vi "[ToBeTest-PC] Continuous Complete Measurament RT.vi"() -> ()   [LabVIEW 2014]
uses:
  <vilib>/FPGAPlugInAG/sbRIO-9636/niLvFpga_Open_sbRIO-9636.vi
  <vilib>/rvi/interface/common/dynamic/niFpgaDynamicAddResources.vi
  <vilib>/FPGAPlugInAG/Dynamic/niLvFpga_Reset_Dynamic.vi
  <vilib>/Utility/error.llb/Error Cluster From Error Code.vi
  <vilib>/rvi/errors/niLvFpgaAdjustHostInterfaceError.vi
  <vilib>/rvi/interface/common/niFpgaWaitOnOcc.vi
  <vilib>/FPGAPlugInAG/Dynamic/niLvFpga_Run_Dynamic.vi
  <vilib>/FPGAPlugInAG/Dynamic/niLvFpga_Abort_Dynamic.vi
  <vilib>/FPGAPlugInAG/Dynamic/niLvFpga_Close_Dynamic.vi
  <vilib>/rvi/interface/nirviOpenFPGA/nirviOpenFPGA.xnode
  FPGA Bitfiles/LaserDistanceSen_FPGATarget_N-ParametricDoub_oZd6Q4K0Aos.lvbitx
  FPGA Target/Test VIs/N-Parametric Double FFT Mesurament (MAX BIN DETECT) SLOW Test.vi
  <vilib>/rvi/interface/nirviMethod/nirviMethod.xnode
  <vilib>/rvi/interface/nirviReadWriteControl/nirviReadWriteControl.xnode
  <vilib>/rvi/interface/nirviCloseFPGA/nirviCloseFPGA.xnode
  <vilib>/rvi/errors/niLvFpgaMergeErrorWithErrorCode.vi
  <vilib>/rvi/interface/Simulation/niFpgaSimulationCallBeginRW.vi
  NiFpgaLv.dll
  <vilib>/Analysis/NI_AALBase.lvlib
  <vilib>/FPGAPlugInAG/Dynamic/niLvFpga_ConfigureFifo_Dynamic.vi
  <vilib>/FPGAPlugInAG/Dynamic/niLvFpga_StartFifo_Dynamic.vi
  <vilib>/FPGAPlugInAG/Dynamic/niLvFpga_ReadFifo_Dynamic.vi
panel:
  out "Standard deviation (m)":dbl format="%0.5f"
  out "cycle time":u32
  out "Distance (m) Plot":dbl(graph)
  in  "#signal for Mean":i32=3000
  out "Relative Standard Deviation":dbl format="%0.7f"
  out "Distance (m)":dbl format="%0.7f"
  in  "stop":bool
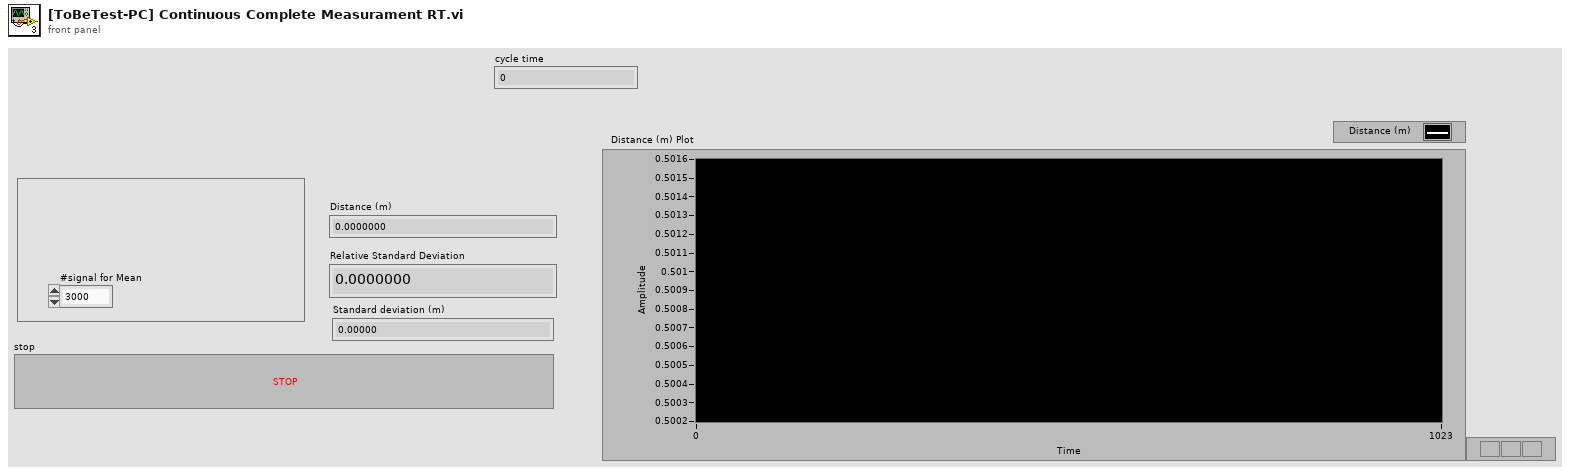
[diagram p1: front panel]
types:
  T1 = enum16{"None", "Hanning", "Hamming", "Blackman", "Blackman-Harris"}
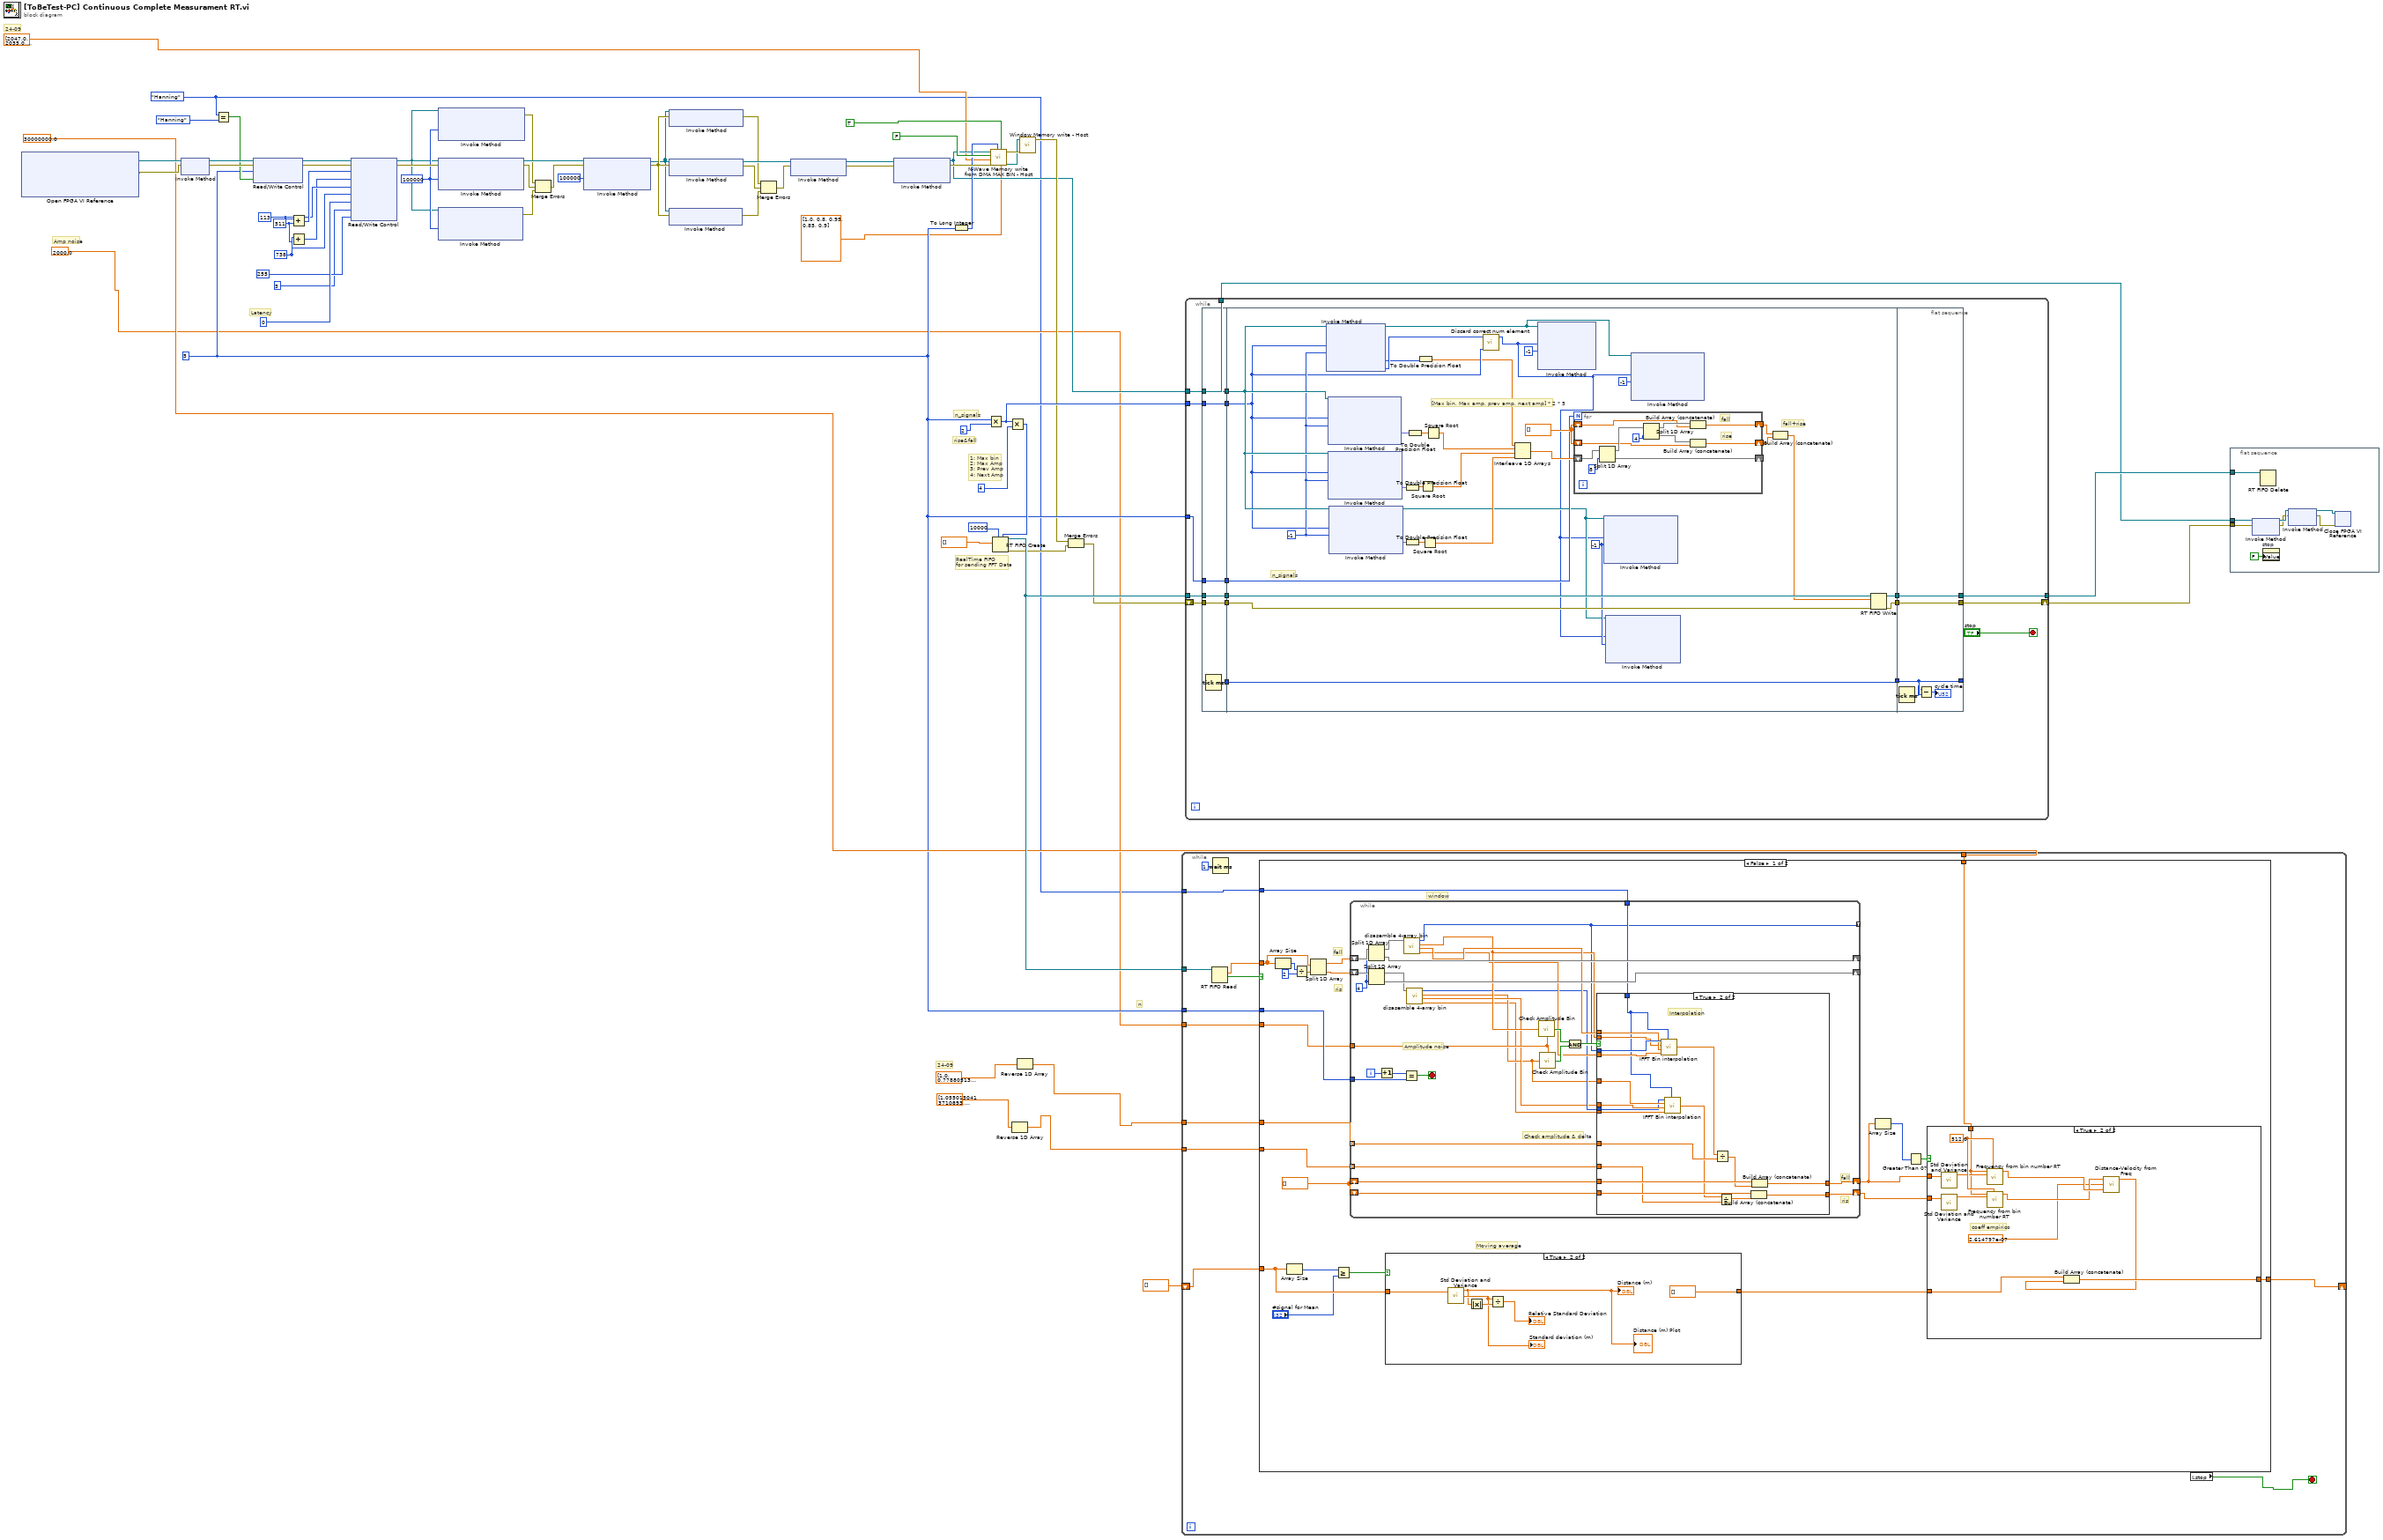
[diagram p0: block diagram]
diagram:
  w6 = T1."Hanning" ("Windowing")
  w62 = u32 738 ("lower limit 2")
  w64 = u32 113 ("lower limit 1")
  w25 = u32 5 ("#Signals")
  w43 = u32 100000 ("Requested Depth")
  w61 = u32 511 ("y")
  # "24-09"
  # "Latency"
  # "24-09"
  # "Amp noise"
  # "n_signals"
  # "rise&fall"
  # "1: Max bin\n2: Max Amp\n3: Prev Amp\n4: Next Amp"
  # "n"
  # "RealTime FIFO \nfor sending FFT Data"
  n1 = xnode "Open FPGA VI Reference"() -> ("FPGA VI Reference Out"=w56:refnum<k20>, "error out"=w55:errorcluster)  [unwired: 2 in]
  n2 = xnode "Invoke Method"("FPGA VI Reference In"=w56, "error in"=w55) -> ("FPGA VI Reference Out"=w53:refnum<k20>, "error out"=w54:errorcluster)
  n3 = Equal?(x=w6, y=T1."Hanning" ("Windowing")) -> (x = y?=w46:bool)
  n4 = xnode "Read/Write Control"("FPGA VI Reference In"=w53, "error in"=w54, "n"=w25, "Hanning window"=w46) -> ("FPGA VI Reference Out"=w52:refnum<k20>, "error out"=w51:errorcluster)
  n5 = Add(x=w64, y=w61) -> (x+y=w65:u32)
  n6 = Add(x=w62, y=w61) -> (x+y=w63:u32)
  n7 = xnode "Read/Write Control"("FPGA VI Reference In"=w52, "error in"=w51, "upper limit 1"=w65, "upper limit 2"=w63, "lower limit 1"=w64, "lower limit 2"=w62, "Latency points"=u32 0 ("Initial Latency points"), "First bin"=5 ("first bin"), "Last bin"=255 ("last bin")) -> ("FPGA VI Reference Out"=w23:refnum<k20>, "error out"=w60:errorcluster)
  n8 = xnode "Invoke Method"("FPGA VI Reference In"=w23, "Requested Depth"=w43) -> ("error out"=w42:errorcluster)  [unwired: 1 in, 2 out]
  n9 = xnode "Invoke Method"("FPGA VI Reference In"=w23, "error in"=w60, "Requested Depth"=w43) -> ("FPGA VI Reference Out"=w57:refnum<k20>, "error out"=w41:errorcluster)  [unwired: 1 out]
  n10 = xnode "Invoke Method"("FPGA VI Reference In"=w23, "Requested Depth"=w43) -> ("error out"=w40:errorcluster)  [unwired: 1 in, 2 out]
  n11 = Merge Errors(w42, w41, w40) -> (w39:errorcluster)
  n12 = xnode "Invoke Method"("FPGA VI Reference In"=w57, "error in"=w39, "Requested Depth"=u32 100000) -> ("FPGA VI Reference Out"=w31:refnum<k20>, "error out"=w32:errorcluster)  [unwired: 1 out]
  n13 = xnode "Invoke Method"("FPGA VI Reference In"=w31, "error in"=w32) -> ("error out"=w30:errorcluster)  [unwired: 1 out]
  n14 = xnode "Invoke Method"("FPGA VI Reference In"=w31, "error in"=w32) -> ("FPGA VI Reference Out"=w35:refnum<k20>, "error out"=w36:errorcluster)
  n15 = xnode "Invoke Method"("FPGA VI Reference In"=w31, "error in"=w32) -> ("error out"=w37:errorcluster)  [unwired: 1 out]
  n16 = Merge Errors(w30, w36, w37) -> (w38:errorcluster)
  n17 = xnode "Invoke Method"("FPGA VI Reference In"=w35, "error in"=w38) -> ("FPGA VI Reference Out"=w34:refnum<k20>, "error out"=w33:errorcluster)
  n18 = xnode "Invoke Method"("FPGA VI Reference In"=w34, "error in"=w33) -> ("FPGA VI Reference Out"=w10:refnum<k20>, "error out"=w15:errorcluster)  [unwired: 1 in]
  n19 = To Long Integer(number=w25) -> (32bit integer=w12:i32)
  n20 = Multiply(x=w25, y=u32 2 ("elements in array (1)")) -> (x*y=w26:u32)
  n21 = call "N-Wave Memory write from DMA MAX BIN - Host.vi"("Triangular Multiply Factor"=dbl[] [1.0, 0.8, 0.95, 0.85, 0.9], "Enable triangular scaling"=TRUE, "n"=w12, "error in"=w15, "Custom Triangular Signal (fal-ris)"=dbl[] [2047.0, 2035.0, 2022.0, 2010.0, 1997.0, 1985.0, 1972.0, 1960.0, 1948.0, 1935.0, 1923.0, 1911.0, 1899.0, 1886.0, 1874.0, 1862.0, 1850.0, 1838.0, 1825.0, 1813.0, 1801.0, 1789.0, 1777.0, 1765.0, 1753.0, 1741.0, 1729.0, 1717.0, 1705.0, 1693.0, 1681.0, 1669.0, 1657.0, 1645.0, 1634.0, 1622.0, 1610.0, 1598.0, 1586.0, 1575.0, 1563.0, 1551.0, 1540.0, 1528.0, 1516.0, 1505.0, 1493.0, 1481.0, 1470.0, 1458.0, 1447.0, 1435.0, 1424.0, 1412.0, 1401.0, 1389.0, 1378.0, 1366.0, 1355.0, 1344.0, 1332.0, 1321.0, 1310.0, 1298.0, 1287.0, 1276.0, 1265.0, 1253.0, 1242.0, 1231.0, 1220.0, 1209.0, 1198.0, 1186.0, 1175.0, 1164.0, 1153.0, 1142.0, 1131.0, 1120.0, 1109.0, 1098.0, 1087.0, 1076.0, 1065.0, 1055.0, 1044.0, 1033.0, 1022.0, 1011.0, 1000.0, 990.0, 979.0, 968.0, 958.0, 947.0, 936.0, 926.0, 915.0, 904.0, 894.0, 883.0, 873.0, 862.0, 852.0, 841.0, 831.0, 820.0, 810.0, 799.0, 789.0, 778.0, 768.0, 758.0, 747.0, 738.0, 727.0, 719.0, 712.0, 706.0, 700.0, 693.0, 687.0, 680.0, 674.0, 668.0, 661.0, 655.0, 648.0, 642.0, 636.0, 629.0, 623.0, 617.0, 610.0, 604.0, 598.0, 591.0, 584.0, 577.0, 569.0, 560.0, 552.0, 545.0, 538.0, 531.0, 525.0, 519.0, 512.0, 506.0, 500.0, 494.0, 488.0, 482.0, 476.0, 470.0, 464.0, 458.0, 452.0, 446.0, 436.0, 430.0, 424.0, 418.0, 412.0, 406.0, 400.0, 394.0, 388.0, 382.0, 376.0, 370.0, 364.0, 358.0, 352.0, 346.0, 338.0, 332.0, 325.0, 319.0, 313.0, 307.0, 301.0, 295.0, 290.0, 284.0, 278.0, 272.0, 267.0, 261.0, 255.0, 249.0, 244.0, 238.0, 232.0, 227.0, 221.0, 215.0, 209.0, 204.0, 198.0, 192.0, 187.0, 181.0, 175.0, 170.0, 164.0, 158.0, 153.0, 147.0, 141.0, 136.0, 130.0, 124.0, 119.0, 113.0, 108.0, 102.0, 96.0, 91.0, 85.0, 79.0, 74.0, 68.0, 62.0, 57.0, 51.0, 45.0, 39.0, 34.0, 28.0, 22.0, 16.0, 11.0, 5.0, 0.0, -6.0, -11.0, -17.0, -22.0, -28.0, -33.0, -39.0, -44.0, -50.0, -55.0, -61.0, -66.0, -72.0, -77.0, -83.0, -88.0, -94.0, -99.0, -105.0, -110.0, -116.0, -121.0, -127.0, -132.0, -137.0, -143.0, -148.0, -154.0, -159.0, -165.0, -170.0, -176.0, -181.0, -186.0, -192.0, -197.0, -203.0, -208.0, -214.0, -219.0, -224.0, -230.0, -235.0, -241.0, -246.0, -251.0, -257.0, -262.0, -268.0, -273.0, -278.0, -284.0, -289.0, -295.0, -300.0, -305.0, -311.0, -316.0, -321.0, -327.0, -332.0, -337.0, -343.0, -348.0, -354.0, -359.0, -364.0, -370.0, -375.0, -380.0, -386.0, -391.0, -397.0, -402.0, -407.0, -413.0, -418.0, -423.0, -429.0, -434.0, -439.0, -445.0, -450.0, -455.0, -461.0, -466.0, -471.0, -477.0, -482.0, -487.0, -493.0, -498.0, -503.0, -509.0, -514.0, -519.0, -525.0, -530.0, -535.0, -540.0, -546.0, -551.0, -556.0, -562.0, -567.0, -572.0, -578.0, -583.0, -588.0, -593.0, -599.0, -604.0, -609.0, -615.0, -620.0, -625.0, -630.0, -636.0, -641.0, -646.0, -651.0, -657.0, -662.0, -667.0, -673.0, -678.0, -683.0, -688.0, -694.0, -699.0, -704.0, -709.0, -715.0, -720.0, -725.0, -730.0, -736.0, -741.0, -746.0, -751.0, -757.0, -762.0, -767.0, -772.0, -778.0, -783.0, -788.0, -793.0, -799.0, -804.0, -809.0, -814.0, -820.0, -825.0, -830.0, -835.0, -841.0, -846.0, -851.0, -856.0, -862.0, -867.0, -872.0, -877.0, -883.0, -888.0, -893.0, -898.0, -903.0, -909.0, -914.0, -919.0, -924.0, -930.0, -935.0, -940.0, -945.0, -951.0, -956.0, -961.0, -966.0, -971.0, -977.0, -982.0, -987.0, -992.0, -998.0, -1003.0, -1008.0, -1013.0, -1018.0, -1024.0, -1029.0, -1034.0, -1039.0, -1045.0, -1050.0, -1055.0, -1060.0, -1065.0, -1071.0, -1076.0, -1081.0, -1086.0, -1092.0, -1097.0, -1102.0, -1107.0, -1112.0, -1118.0, -1123.0, -1128.0, -1133.0, -1138.0, -1144.0, -1149.0, -1154.0, -1159.0, -1165.0, -1170.0, -1175.0, -1180.0, -1185.0, -1191.0, -1196.0, -1201.0, -1206.0, -1211.0, -1217.0, -1222.0, -1227.0, -1232.0, -1237.0, -1243.0, -1248.0, -1253.0, -1258.0, -1263.0, -1269.0, -1274.0, -1279.0, -1284.0, -1289.0, -1295.0, -1300.0, -1305.0, -1310.0, -1315.0, -1321.0, -1326.0, -1331.0, -1336.0, -1341.0, -1347.0, -1352.0, -1357.0, -1362.0, -1367.0, -1373.0, -1378.0, -1383.0, -1388.0, -1393.0, -1399.0, -1404.0, -1409.0, -1414.0, -1419.0, -1425.0, -1430.0, -1435.0, -1440.0, -1445.0, -1450.0, -1456.0, -1461.0, -1466.0, -1471.0, -1476.0, -1482.0, -1487.0, -1492.0, -1497.0, -1502.0, -1508.0, -1513.0, -1518.0, -1523.0, -1528.0, -1534.0, -1539.0, -1544.0, -1549.0, -1554.0, -1560.0, -1565.0, -1570.0, -1575.0, -1580.0, -1586.0, -1591.0, -1596.0, -1601.0, -1606.0, -1612.0, -1617.0, -1622.0, -1627.0, -1632.0, -1637.0, -1643.0, -1648.0, -1653.0, -1658.0, -1663.0, -1669.0, -1674.0, -1679.0, -1684.0, -1689.0, -1695.0, -1700.0, -1705.0, -1710.0, -1715.0, -1721.0, -1726.0, -1731.0, -1736.0, -1741.0, -1747.0, -1752.0, -1757.0, -1762.0, -1767.0, -1773.0, -1778.0, -1783.0, -1788.0, -1793.0, -1799.0, -1804.0, -1809.0, -1814.0, -1819.0, -1825.0, -1830.0, -1835.0, -1840.0, -1845.0, -1851.0, -1856.0, -1861.0, -1866.0, -1871.0, -1876.0, -1882.0, -1887.0, -1892.0, -1897.0, -1902.0, -1908.0, -1913.0, -1918.0, -1923.0, -1928.0, -1934.0, -1939.0, -1944.0, -1949.0, -1954.0, -1960.0, -1965.0, -1970.0, -1975.0, -1980.0, -1986.0, -1991.0, -1996.0, -2001.0, -2006.0, -2012.0, -2017.0, -2022.0, -2027.0, -2032.0, -2038.0, -2043.0, -2048.0, -2047.0, -2037.0, -2027.0, -2017.0, -2007.0, -1997.0, -1987.0, -1977.0, -1967.0, -1957.0, -1947.0, -1937.0, -1927.0, -1917.0, -1907.0, -1897.0, -1888.0, -1878.0, -1868.0, -1858.0, -1848.0, -1838.0, -1828.0, -1819.0, -1809.0, -1799.0, -1789.0, -1780.0, -1770.0, -1760.0, -1750.0, -1741.0, -1731.0, -1721.0, -1712.0, -1702.0, -1692.0, -1683.0, -1673.0, -1663.0, -1654.0, -1644.0, -1635.0, -1625.0, -1615.0, -1606.0, -1596.0, -1587.0, -1577.0, -1568.0, -1558.0, -1549.0, -1539.0, -1530.0, -1520.0, -1511.0, -1501.0, -1492.0, -1483.0, -1473.0, -1464.0, -1454.0, -1445.0, -1436.0, -1426.0, -1417.0, -1408.0, -1398.0, -1389.0, -1380.0, -1371.0, -1361.0, -1352.0, -1343.0, -1334.0, -1324.0, -1315.0, -1306.0, -1297.0, -1288.0, -1278.0, -1269.0, -1260.0, -1251.0, -1242.0, -1233.0, -1224.0, -1215.0, -1205.0, -1196.0, -1187.0, -1178.0, -1169.0, -1160.0, -1151.0, -1142.0, -1133.0, -1124.0, -1115.0, -1106.0, -1097.0, -1088.0, -1080.0, -1071.0, -1062.0, -1053.0, -1044.0, -1035.0, -1026.0, -1017.0, -1009.0, -1000.0, -991.0, -982.0, -973.0, -965.0, -953.0, -944.0, -935.0, -920.0, -906.0, -889.0, -871.0, -854.0, -842.0, -834.0, -826.0, -818.0, -810.0, -802.0, -794.0, -786.0, -778.0, -770.0, -762.0, -754.0, -746.0, -739.0, -731.0, -723.0, -715.0, -707.0, -699.0, -690.0, -682.0, -672.0, -661.0, -651.0, -639.0, -627.0, -616.0, -606.0, -598.0, -591.0, -584.0, -577.0, -570.0, -563.0, -556.0, -549.0, -542.0, -535.0, -528.0, -520.0, -513.0, -506.0, -499.0, -492.0, -485.0, -478.0, -471.0, -464.0, -457.0, -451.0, -444.0, -437.0, -430.0, -423.0, -416.0, -409.0, -400.0, -390.0, -382.0, -373.0, -364.0, -356.0, -349.0, -343.0, -336.0, -330.0, -323.0, -317.0, -310.0, -304.0, -297.0, -291.0, -284.0, -278.0, -271.0, -265.0, -258.0, -252.0, -245.0, -239.0, -232.0, -226.0, -219.0, -213.0, -207.0, -200.0, -194.0, -187.0, -181.0, -175.0, -168.0, -162.0, -156.0, -149.0, -143.0, -136.0, -128.0, -121.0, -114.0, -107.0, -100.0, -93.0, -87.0, -80.0, -74.0, -68.0, -62.0, -56.0, -50.0, -44.0, -38.0, -32.0, -26.0, -20.0, -14.0, -8.0, -2.0, 5.0, 11.0, 17.0, 23.0, 29.0, 35.0, 41.0, 47.0, 53.0, 59.0, 65.0, 70.0, 76.0, 82.0, 88.0, 94.0, 100.0, 106.0, 112.0, 118.0, 124.0, 130.0, 136.0, 142.0, 148.0, 154.0, 161.0, 167.0, 174.0, 180.0, 186.0, 192.0, 198.0, 204.0, 210.0, 215.0, 221.0, 227.0, 233.0, 238.0, 244.0, 250.0, 255.0, 261.0, 267.0, 273.0, 278.0, 284.0, 290.0, 295.0, 301.0, 307.0, 312.0, 318.0, 324.0, 329.0, 335.0, 341.0, 346.0, 352.0, 358.0, 363.0, 369.0, 374.0, 380.0, 386.0, 391.0, 397.0, 402.0, 408.0, 414.0, 419.0, 425.0, 430.0, 436.0, 441.0, 447.0, 453.0, 458.0, 464.0, 470.0, 475.0, 481.0, 487.0, 493.0, 499.0, 504.0, 510.0, 516.0, 521.0, 527.0, 532.0, 538.0, 543.0, 549.0, 554.0, 560.0, 565.0, 571.0, 576.0, 582.0, 587.0, 593.0, 598.0, 604.0, 609.0, 614.0, 620.0, 625.0, 631.0, 636.0, 642.0, 647.0, 653.0, 658.0, 663.0, 669.0, 674.0, 680.0, 685.0, 691.0, 696.0, 701.0, 707.0, 712.0, 718.0, 723.0, 728.0, 734.0, 739.0, 745.0, 750.0, 755.0, 761.0, 766.0, 772.0, 777.0, 782.0, 788.0, 793.0, 798.0, 804.0, 809.0, 815.0, 820.0, 826.0, 831.0, 837.0, 842.0, 847.0, 853.0, 858.0, 863.0, 869.0, 874.0, 880.0, 885.0, 890.0, 895.0, 901.0, 906.0, 911.0, 917.0, 922.0, 927.0, 933.0, 938.0, 943.0, 948.0, 954.0, 959.0, 964.0, 970.0, 975.0, 980.0, 985.0, 991.0, 996.0, 1001.0, 1006.0, 1012.0, 1017.0, 1022.0, 1027.0, 1033.0, 1038.0, 1043.0, 1048.0, 1054.0, 1059.0, 1064.0, 1069.0, 1075.0, 1080.0, 1085.0, 1090.0, 1096.0, 1101.0, 1106.0, 1111.0, 1116.0, 1122.0, 1127.0, 1132.0, 1137.0, 1143.0, 1148.0, 1153.0, 1158.0, 1163.0, 1169.0, 1174.0, 1179.0, 1184.0, 1190.0, 1195.0, 1200.0, 1205.0, 1211.0, 1216.0, 1221.0, 1226.0, 1231.0, 1237.0, 1242.0, 1247.0, 1252.0, 1257.0, 1262.0, 1268.0, 1273.0, 1278.0, 1283.0, 1288.0, 1293.0, 1298.0, 1304.0, 1309.0, 1314.0, 1319.0, 1324.0, 1329.0, 1334.0, 1340.0, 1345.0, 1350.0, 1355.0, 1360.0, 1365.0, 1370.0, 1375.0, 1381.0, 1386.0, 1391.0, 1396.0, 1401.0, 1406.0, 1411.0, 1416.0, 1421.0, 1427.0, 1432.0, 1437.0, 1442.0, 1447.0, 1452.0, 1457.0, 1462.0, 1467.0, 1472.0, 1478.0, 1483.0, 1488.0, 1493.0, 1498.0, 1503.0, 1508.0, 1513.0, 1518.0, 1523.0, 1528.0, 1534.0, 1539.0, 1544.0, 1549.0, 1554.0, 1559.0, 1564.0, 1569.0, 1574.0, 1579.0, 1584.0, 1589.0, 1595.0, 1600.0, 1605.0, 1610.0, 1615.0, 1620.0, 1625.0, 1630.0, 1635.0, 1640.0, 1645.0, 1650.0, 1655.0, 1660.0, 1666.0, 1671.0, 1676.0, 1681.0, 1686.0, 1691.0, 1696.0, 1701.0, 1706.0, 1711.0, 1716.0, 1721.0, 1726.0, 1731.0, 1736.0, 1741.0, 1746.0, 1751.0, 1757.0, 1762.0, 1767.0, 1772.0, 1777.0, 1782.0, 1787.0, 1792.0, 1797.0, 1802.0, 1807.0, 1812.0, 1817.0, 1822.0, 1827.0, 1832.0, 1837.0, 1842.0, 1847.0, 1852.0, 1857.0, 1862.0, 1867.0, 1872.0, 1877.0, 1883.0, 1888.0, 1893.0, 1898.0, 1903.0, 1908.0, 1913.0, 1918.0, 1923.0, 1928.0, 1933.0, 1938.0, 1943.0, 1948.0, 1953.0, 1958.0, 1963.0, 1968.0, 1973.0, 1978.0, 1983.0, 1988.0, 1993.0, 1998.0, 2003.0, 2008.0, 2013.0, 2018.0, 2023.0, 2028.0, 2033.0, 2038.0, 2043.0, 2048.0] ("appended array"), "Triangolo dritto?"=FALSE, "FPGA VI Reference In"=w10) -> ("FPGA VI Reference Out"=w11:refnum<k20>, "error out"=w16:errorcluster)  [unwired: 2 in, 1 out]
  n22 = Multiply(x=w26, y=u32 4 ("elements in array (1)")) -> (x*y=w27:u32)
  n23 = RT FIFO Create(1:dbl[] [] ("first subarray"), 4:u32 10000 ("size (10)"), 6:w27) -> (8:w49:refnum<k33>, 11:w19:errorcluster)  [unwired: 5 in, 1 out]
  n24 = Reverse 1D Array(array=dbl[] [1.0550150413710893, 0.8807744280543515, 1.0096480344577006, 0.9233799836458207, 0.9653106595082892] ("mean factor 2")) -> (reversed array=w1:dbl[])
  n25 = Reverse 1D Array(array=dbl[] [1.0, 0.7788051374952276, 0.9586568902543302, 0.8395566206470091, 0.903068410955916] ("mean factor 1")) -> (reversed array=w3:dbl[])
  n26 = call "Window Memory write - Host.vi"("error in"=w16, "FPGA VI Reference In"=w11) -> ("error out"=w17:errorcluster)  [unwired: 7 in, 2 out]
  n27 = Merge Errors(w17, w19) -> (w18:errorcluster)
  n28 = while {
    tunnel: w49 -> [w78]
    tunnel: w6 -> [w75]
    tunnel: w25 -> [w74]
    shift-right: [w72] -> _
    shift-left: dbl[] [] ("appended array") -> [w73]
    tunnel: 30000000.0 -> [w71]
    tunnel: w3 -> [w70]
    tunnel: w1 -> [w69]
    tunnel: 2000.0 ("Threshold Amp") -> [w68]
    stop <- w66 stop-if-true
    n29 = RT FIFO Read(0:w78) -> (9:w76:dbl[], 10:w77:bool)  [unwired: 3 in, 3 out]
    n30 = Wait (ms)(milliseconds to wait=u32 1) -> ()  [unwired: 1 out]
    n31 = case shown="False" w77 {
      tunnel: w76 -> [w101 _]
      tunnel: w75 -> [w100 _]
      tunnel: w74 -> [w97 _]
      tunnel: w73 -> [w90 w173]
      tunnel: [w88 w173] -> w72
      tunnel: w71 -> [w79 _]
      tunnel: w70 -> [w87 _]
      tunnel: w69 -> [w86 _]
      tunnel: w68 -> [w85 _]
      frame False {
        w96 = dbl[] [] ("appended array")
        # "Moving average"
        # "window"
        # "ris"
        # "fall"
        n32 = Array Size(array=w101) -> (size(s)=w84:i32)
        n33 = Array Size(array=w90) -> (size(s)=w91:i32)
        n34 = Divide(x=w84, y=2) -> (x/y=w82:dbl)
        n35 = Split 1D Array(array=w101, index=w82) -> (first subarray=w98:dbl[], second subarray=w99:dbl[])
        n36 = Greater Or Equal?(x=w91, y="#signal for Mean") -> (x >= y?=w81:bool)
        n37 = while {
          shift-right: [w143] -> _
          shift-left: w98 -> [w151]
          shift-right: [w144] -> _
          shift-left: w99 -> [w150]
          tunnel: w100 -> [w139]
          tunnel: w97 -> [w148]
          shift-right: [w138] -> w95
          shift-left: w96 -> [w136]
          shift-right: [w137] -> w94
          shift-left: w96 -> [w135]
          tunnel: w87 -> [w134] mode=indexing
          tunnel: w86 -> [w133] mode=indexing
          tunnel: w85 -> [w132]
          tunnel: [w122] -> _ mode=indexing
          i -> [w145]
          stop <- w149 stop-if-true
          w147 = 4 ("x")
          # "ris"
          # "fall"
          # "Check amplitude & delta"
          # "Amplitude noise"
          n38 = Split 1D Array(array=w151, index=w147) -> (first subarray=w131:dbl[], second subarray=w143:dbl[])
          n39 = Split 1D Array(array=w150, index=w147) -> (first subarray=w130:dbl[], second subarray=w144:dbl[])
          n40 = Increment(x=w145) -> (x+1=w146:i32)
          n41 = Equal?(x=w146, y=w148) -> (x = y?=w149:bool)
          n42 = call "disasemble 4-array bin.vi"("4-Array Bin-Amp"=w131) -> ("Next Amp"=w127:dbl, "Prev amp"=w129:dbl, "Max amp"=w128:dbl, "Max bin"=w122:i32)  [unwired: 7 in]
          n43 = call "disasemble 4-array bin.vi"("4-Array Bin-Amp"=w130) -> ("Next Amp"=w123:dbl, "Prev amp"=w125:dbl, "Max amp"=w124:dbl, "Max bin"=w126:i32)  [unwired: 7 in]
          n44 = call "Check Amplitude Bin.vi"("Threshold Amp"=w132, "Max Amp"=w128) -> ("Check Amp Ok?"=w142:bool)  [unwired: 2 in]
          n45 = call "Check Amplitude Bin.vi"("Threshold Amp"=w132, "Max Amp"=w124) -> ("Check Amp Ok?"=w141:bool)  [unwired: 2 in]
          n46 = And(x=w142, y=w141) -> (x .and. y?=w140:bool)
          n47 = case shown="True" w140 {
            tunnel: w125 -> [_ w172]
            tunnel: w123 -> [_ w171]
            tunnel: w124 -> [_ w170]
            tunnel: w126 -> [_ w169]
            tunnel: w122 -> [_ w168]
            tunnel: w129 -> [_ w167]
            tunnel: w128 -> [_ w166]
            tunnel: w127 -> [_ w165]
            tunnel: w139 -> [_ w164]
            tunnel: [w153 w159] -> w138
            tunnel: [w152 w158] -> w137
            tunnel: w136 -> [w153 w163]
            tunnel: w135 -> [w152 w162]
            tunnel: w134 -> [_ w161]
            tunnel: w133 -> [_ w160]
            frame False {
            }
            frame True {
              # "Interpolation"
              n48 = call "IFFT Bin interpolation.vi"("Max Bin"=w168, "Max Amp"=w166, "Prev Max Amp"=w167, "Succ Max Amp"=w165, "Windowing"=w164) -> ("Interpolate Bin"=w157:dbl)
              n49 = call "IFFT Bin interpolation.vi"("Max Bin"=w169, "Max Amp"=w170, "Prev Max Amp"=w172, "Succ Max Amp"=w171, "Windowing"=w164) -> ("Interpolate Bin"=w156:dbl)
              n50 = Divide(x=w157, y=w161) -> (x/y=w155:dbl)
              n51 = Divide(x=w156, y=w160) -> (x/y=w154:dbl)
              n52 = Build Array (concatenate)(w162, w154) -> (w158:dbl[])
              n53 = Build Array (concatenate)(w163, w155) -> (w159:dbl[])
            }
          }
        }
        n54 = case shown="True" w81 {
          tunnel: w90 -> [w102 w107]
          tunnel: [w102 dbl[] [] ("appended array")] -> w89
          frame False {
          }
          frame True {
            n55 = call <vilib>:"Std Deviation and Variance.vi"("X"=w107) -> ("mean"=w103:dbl, "standard deviation"=w105:dbl)  [unwired: 1 in, 1 out]
            "Distance (m)" <- w103
            "Distance (m) Plot" <- w103
            "Standard deviation (m)" <- w105
            n56 = Absolute Value(x=w103) -> (abs(x)=w108:dbl)
            n57 = Divide(x=w105, y=w108) -> (x/y=→"Relative Standard Deviation":dbl)
          }
        }
        n58 = Array Size(array=w95) -> (size(s)=w93:i32)
        n59 = Greater Than 0?(x=w93) -> (x > 0?=w92:bool)
        n60 = case shown="True" w92 {
          tunnel: w95 -> [_ w120]
          tunnel: w94 -> [_ w119]
          tunnel: w89 -> [w109 w114]
          tunnel: [w109 w113] -> w88
          tunnel: w79 -> [_ w112]
          frame False {
          }
          frame True {
            w121 = 512.0 ("FFT size")
            # "coeff empirico"
            n61 = call <vilib>:"Std Deviation and Variance.vi"("X"=w120) -> ("mean"=w115:dbl)  [unwired: 1 in, 2 out]
            n62 = call <vilib>:"Std Deviation and Variance.vi"("X"=w119) -> ("mean"=w116:dbl)  [unwired: 1 in, 2 out]
            n63 = call "Frequency from bin number RT.vi"("FFT size"=w121, "Bin number"=w115, "Sample Rate (S/s)"=w112) -> ("Detected Frequency (Hz)"=w118:dbl)  [unwired: 8 in]
            n64 = call "Frequency from bin number RT.vi"("FFT size"=w121, "Bin number"=w116, "Sample Rate (S/s)"=w112) -> ("Detected Frequency (Hz)"=w117:dbl)  [unwired: 8 in]
            n65 = call "Distance-Velocity from Freq.vi"("freq_rising"=w117, "Empirical Distance Costant"=2.614797e-07, "freq_falling"=w118) -> ("Distance (m)"=w111:dbl)  [unwired: 2 in, 2 out]
            n66 = Build Array (concatenate)(w114, w111) -> (w113:dbl[])
          }
        }
      }
      frame True {
      }
    }
    n67 = local read "stop"() -> (w66:bool)
  }
  n68 = while {
    tunnel: w10 -> [w185]
    tunnel: w49 -> [w190]
    tunnel: w26 -> [w183]
    shift-right: [w188] -> w22
    shift-left: w18 -> [w189]
    tunnel: w25 -> [w187]
    tunnel: [w186] -> w21
    tunnel: [w185] -> w20
    stop <- "stop" stop-if-true
    n69 = flat-sequence {
      tunnel: w183 -> [w192]
      tunnel: w185 -> [w193]
      tunnel: w187 -> [w194]
      tunnel: w189 -> [w195]
      tunnel: w190 -> [w196]
      tunnel: [w196] -> w182
      tunnel: [w195] -> w181
      tunnel: [w194] -> w180
      tunnel: [w193] -> w179
      tunnel: [w192] -> w178
      tunnel: [w191] -> w177
      tunnel: w182 -> [w228]
      tunnel: w181 -> [w227]
      tunnel: w180 -> [w218]
      tunnel: w179 -> [w210]
      tunnel: w178 -> [w201]
      tunnel: w177 -> [w198]
      tunnel: [w223] -> w176
      tunnel: [w211] -> w175
      tunnel: [w198] -> w174
      tunnel: [w241] -> _
      tunnel: [w243] -> w186
      tunnel: [w244] -> w188
      tunnel: w176 -> [w244]
      tunnel: w175 -> [w243]
      tunnel: w174 -> [w241]
      frame #0 {
        n70 = Tick Count (ms)() -> (millisecond timer value=w191:u32)
      }
      frame #1 {
        w205 = -1 ("Timeout (ms)")
        w222 = dbl[] [] ("first subarray")
        w202 = -1 ("Timeout (ms)")
        # "n_signals"
        # "fall+rise"
        # "[Max bin, Max amp, prev amp, next amp] * 2 * 5"
        n71 = xnode "Invoke Method"("FPGA VI Reference In"=w210, "Number of Elements"=w201, "Timeout (ms)"=w202) -> ("FPGA VI Reference Out"=w206:refnum<k20>, "Data"=w200:i32[], "Elements Remaining"=w203:u32)  [unwired: 1 in, 1 out]
        n72 = xnode "Invoke Method"("FPGA VI Reference In"=w210, "Number of Elements"=w201, "Timeout (ms)"=w202) -> ("Data"=w217:fxp<+,44,44>[])  [unwired: 1 in, 3 out]
        n73 = xnode "Invoke Method"("FPGA VI Reference In"=w210, "Number of Elements"=w201, "Timeout (ms)"=w202) -> ("Data"=w215:fxp<+,44,44>[])  [unwired: 1 in, 3 out]
        n74 = xnode "Invoke Method"("FPGA VI Reference In"=w210, "Number of Elements"=w201, "Timeout (ms)"=w202) -> ("FPGA VI Reference Out"=w204:refnum<k20>, "Data"=w213:fxp<+,44,44>[])  [unwired: 1 in, 2 out]
        n75 = To Double Precision Float(number=w215) -> (double precision float=w214:dbl[])
        n76 = To Double Precision Float(number=w213) -> (double precision float=w212:dbl[])
        n77 = To Double Precision Float(number=w217) -> (double precision float=w216:dbl[])
        n78 = To Double Precision Float(number=w200) -> (double precision float=w199:dbl[])
        n79 = Square Root(x=w214) -> (sqrt(x)=w225:dbl[])
        n80 = Square Root(x=w212) -> (sqrt(x)=w224:dbl[])
        n81 = Square Root(x=w216) -> (sqrt(x)=w226:dbl[])
        n82 = call "Discard correct num element.vi"("Read packet dim"=w201, "Element Remaing in Queue"=w203) -> ("Effective read element"=w197:i32)  [unwired: 9 in]
        n83 = Interleave 1D Arrays(w199, w226, w225, w224) -> (w219:dbl[])
        n84 = xnode "Invoke Method"("FPGA VI Reference In"=w206, "Number of Elements"=w197, "Timeout (ms)"=-1) -> ()  [unwired: 1 in, 4 out]
        n85 = for {
          N: w218 -> [_]
          shift-right: [w237] -> _
          shift-left: w219 -> [w239]
          shift-right: [w231] -> w221
          shift-left: w222 -> [w232]
          shift-right: [w229] -> w220
          shift-left: w222 -> [w230]
          # "rise"
          # "fall"
          n86 = Split 1D Array(array=w239, index=8) -> (first subarray=w236:dbl[], second subarray=w237:dbl[])
          n87 = Split 1D Array(array=w236, index=4) -> (first subarray=w233:dbl[], second subarray=w234:dbl[])
          n88 = Build Array (concatenate)(w233, w232) -> (w231:dbl[])
          n89 = Build Array (concatenate)(w234, w230) -> (w229:dbl[])
        }
        n90 = xnode "Invoke Method"("FPGA VI Reference In"=w204, "Number of Elements"=w197, "Timeout (ms)"=w205) -> ()  [unwired: 1 in, 4 out]
        n91 = xnode "Invoke Method"("FPGA VI Reference In"=w204, "Number of Elements"=w197, "Timeout (ms)"=w205) -> ()  [unwired: 1 in, 4 out]
        n92 = xnode "Invoke Method"("FPGA VI Reference In"=w206, "Number of Elements"=w197, "Timeout (ms)"=-1) -> ()  [unwired: 1 in, 4 out]
        n93 = Build Array (concatenate)(w221, w220) -> (w209:dbl[])
        n94 = RT FIFO Write(0:w228, 1:w209, 3:w227) -> (8:w211:refnum<k33>, 11:w223:errorcluster)  [unwired: 2 in, 2 out]
      }
      frame #2 {
        n95 = Tick Count (ms)() -> (millisecond timer value=w240:u32)
        n96 = Subtract(x=w240, y=w241) -> (x-y=→"cycle time":u32)
      }
    }
  }
  n97 = flat-sequence {
    tunnel: w22 -> [w252]
    tunnel: w20 -> [w247]
    tunnel: w21 -> [w245]
    frame #0 {
      n98 = xnode "Invoke Method"("FPGA VI Reference In"=w247, "error in"=w252) -> ("FPGA VI Reference Out"=w249:refnum<k20>, "error out"=w248:errorcluster)
      n99 = RT FIFO Delete(0:w245) -> ()  [unwired: 2 in, 1 out]
      n100 = property on="stop" class="Bool (strict)"("Value"=FALSE ("stop")) -> ()  [unwired: 2 in, 2 out]
      n101 = xnode "Invoke Method"("FPGA VI Reference In"=w249, "error in"=w248) -> ("FPGA VI Reference Out"=w250:refnum<k20>, "error out"=w251:errorcluster)
      n102 = xnode "Close FPGA VI Reference"("FPGA VI Reference In"=w250, "error in"=w251) -> ()  [unwired: 1 out]
    }
  }
